vi "process safe state.vi"(8 "error in":errorcluster, 9 "result allocation":T1, 10 "parameters":T1, 11 "Temperature Chamber Model runtime in":refnum<class "Temperature Chamber Model runtime.lvclass">) -> (0 "error out":errorcluster, 1 "results":T1, 2 "parameter allocation":T1, 3 "Temperature Chamber Model runtime out":refnum<class "Temperature Chamber Model runtime.lvclass">)   [LabVIEW 2015, in "Temperature Chamber Model runtime.lvclass"]
doc: "Provides an interface for information processing by a module when in a safe state. This interface simply calls the normal processing function. However, if child modules need to have custom logic during safe-state operation, this can be implemented here.\nNI Tag Bus Module Framework 1.0.2.34\nNI Systems Engineering"
uses:
  Temperature Chamber Model runtime.lvclass
  <vilib>/NI/Tag Bus/table/data table.ctl
  <vilib>/NI/Tag Bus/table/data table.lvlib
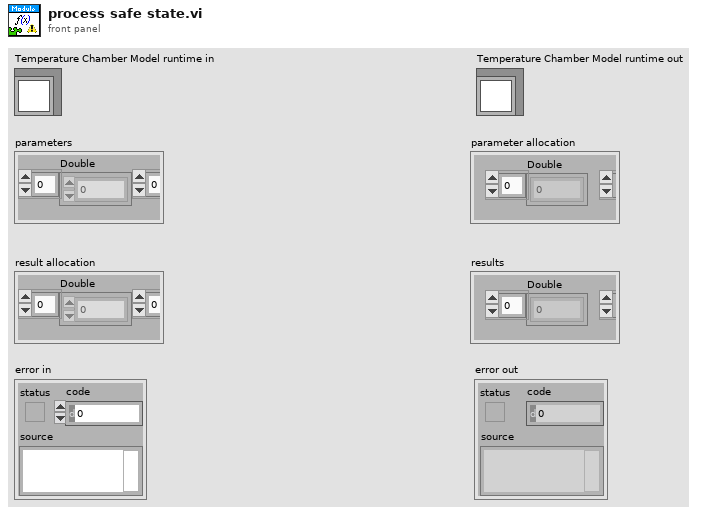
[diagram p1: front panel]
types:
  T1 = typedef "tag bus.lvlib/data table.lvlib/data table.ctl" = cluster{"Double":dbl[], "Single":sgl[], "I64":i64[], "I32":i32[], "I16":i16[], "I8":i8[], "U64":u64[], "U32":u32[], "U16":u16[], "U8":u8[], "Boolean":bool[], "String":string[], "Array of Double":cluster{"DBL Array":dbl[]}[], "Array of Single":cluster{"SGL Array":sgl[]}[], "Array of I64":cluster{"I64 Array":i64[]}[], "Array of I32":cluster{"I32 Array":i32[]}[], "Array of I16":cluster{"I16 Array":i16[]}[], "Array of I8":cluster{"I8 Array":i8[]}[], "Array of U64":cluster{"U64 Array":u64[]}[], "Array of U32":cluster{"U32 Array":u32[]}[], "Array of U16":cluster{"U16 Array":u16[]}[], "Array of U8":cluster{"U8 Array":u8[]}[], "Array of Boolean":cluster{"Boolean Array":bool[]}[], "Array of String":cluster{"String Array":string[]}[]}
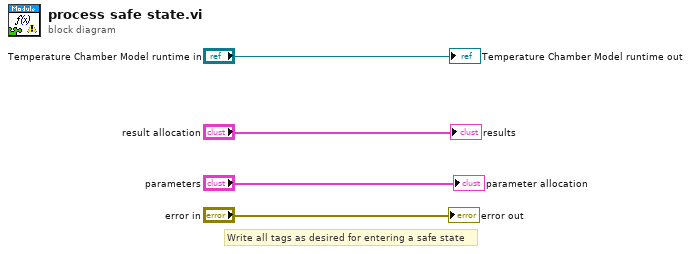
[diagram p0: block diagram]
diagram:
  # "Write all tags as desired for entering a safe state"
  "Temperature Chamber Model runtime out" <- "Temperature Chamber Model runtime in"
  "error out" <- "error in"
  "results" <- "result allocation"
  "parameter allocation" <- "parameters"
